vi "Manual Override Loop.vi"(0 "Current Valve State Array":refnum<vi>, 2 "Manual Valve Array":refnum<vi>[](array[refnum]), 4 "Stop Process":refnum<vi>, 6 "System Queue":refnum<vi>, 7 "N2 Valves":i32[](array[numeric]), 8 "JSON Queue":refnum<vi>, 9 "Pump Valves":i32[](array[numeric]), 10 "Locks (-)":refnum<vi>, 11 "Valves Per Reactor":i32, 12 "Debug Mode":refnum<vi>, 13 "Number of Reactors":i32, 14 "Reactor Name":string, 15 "Reactor Selector":T1(ring), 19 "Number of Shared Lines":i32) -> ()   [LabVIEW 2021]
uses:
  a8b2c1af-05a2-43ad-9eca-c9421cccccff.vi
  <vilib>/Comparison/Equal/Equal Functor/Equal Functor.lvclass
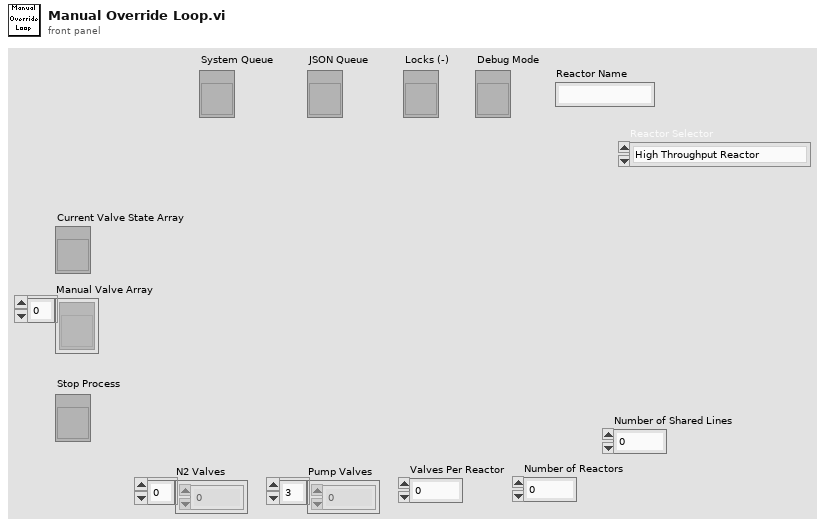
[diagram p1: front panel]
types:
  T1 = enum16{"High Throughput Reactor", "In Situ Reactor", "MLD Reactor"}
  T2 = enum16{"Lock", "Release", "Check", "Check All", "Release All"}
  T3 = enum8{"Enabled", "Disabled", "Disabled and Grayed Out"}
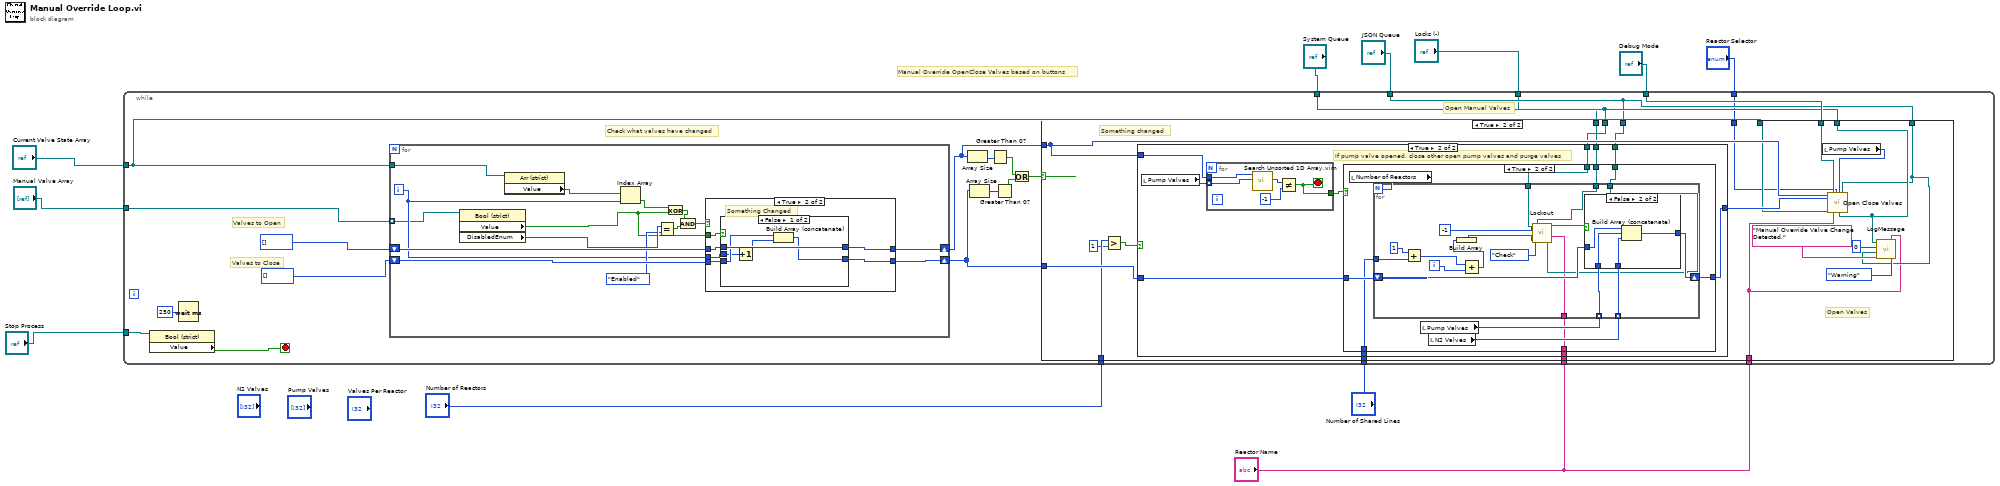
[diagram p0: block diagram]
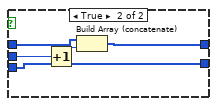
[diagram p7: hidden frame]
diagram:
  # "Manual Override OpenClose Valves based on buttons"
  n1 = while {
    tunnel: "Current Valve State Array" -> [w21]
    tunnel: "Stop Process" -> [w24]
    tunnel: "Debug Mode" -> [w22]
    tunnel: "System Queue" -> [w20]
    tunnel: "JSON Queue" -> [w19]
    tunnel: "Locks (-)" -> [w18]
    tunnel: "Manual Valve Array" -> [w17]
    tunnel: "Number of Reactors" -> [w16]
    tunnel: "Number of Shared Lines" -> [w15]
    tunnel: "Reactor Name" -> [w14]
    tunnel: "Reactor Name" -> [w13]
    tunnel: "Reactor Selector" -> [w12]
    stop <- w23 stop-if-true
    # "Open Manual Valves"
    # "Check what valves have changed"
    # "Valves to Open"
    # "Valves to Close"
    n2 = property class="Bool (strict)"(reference=w24) -> ("Value"=w23:bool)  [unwired: 1 in, 2 out]
    n3 = Wait (ms)(milliseconds to wait=u32 250 ("millisecond multiple")) -> ()  [unwired: 1 out]
    n4 = for {
      tunnel: w17 -> [w105] mode=indexing
      shift-right: [w118] -> w26
      shift-left: i32[] [] -> [w119]
      shift-right: [w116] -> w25
      shift-left: i32[] [] -> [w117]
      tunnel: w21 -> [w107]
      i -> [w108]
      n5 = property class="Bool (strict)"(reference=w105) -> ("Value"=w106:bool, "DisabledEnum"=w114:T3)  [unwired: 1 in, 2 out]
      n6 = property class="Arr (strict)"(reference=w107) -> ("Value"=w109:bool[])  [unwired: 1 in, 2 out]
      n7 = Index Array(array=w109, index=w108) -> (element=w115:bool)
      n8 = Equal?(x=w114, y=T3."Enabled") -> (x = y?=w110:bool)
      n9 = Exclusive Or(1:w106, 2:w115) -> (0:w111:bool)
      n10 = And(x=w111, y=w110) -> (x .and. y?=w112:bool)
      n11 = case shown="True" w112 {
        tunnel: w106 -> [_ w127]
        tunnel: w119 -> [w121 w126]
        tunnel: [w121 w125] -> w118
        tunnel: w108 -> [_ w124]
        tunnel: w117 -> [w120 w123]
        tunnel: [w120 w122] -> w116
        frame False {
        }
        frame True {
          # "Something Changed"
          n12 = case shown="False" w127 {
            tunnel: w126 -> [w132 w137]
            tunnel: [w132 w136] -> w125
            tunnel: w124 -> [w130 w135]
            tunnel: w123 -> [w131 w134]
            tunnel: [w129 w134] -> w122
            frame False {
              n13 = Increment(x=w130) -> (x+1=w128:i32)
              n14 = Build Array (concatenate)(w131, w128) -> (w129:i32[])
            }
            frame True {
              n15 = Increment(x=w135) -> (x+1=w133:i32)
              n16 = Build Array (concatenate)(w137, w133) -> (w136:i32[])
            }
          }
        }
      }
    }
    n17 = Array Size(array=w26) -> (size(s)=w32:i32)
    n18 = Array Size(array=w25) -> (size(s)=w29:i32)
    n19 = Greater Than 0?(x=w32) -> (x > 0?=w30:bool)
    n20 = Greater Than 0?(x=w29) -> (x > 0?=w28:bool)
    n21 = Or(x=w30, y=w28) -> (x .or. y?=w31:bool)
    n22 = case shown="True" w31 {
      tunnel: w26 -> [_ w54]
      tunnel: w25 -> [_ w53]
      tunnel: w22 -> [_ w48]
      tunnel: w20 -> [_ w47]
      tunnel: w19 -> [_ w46]
      tunnel: w21 -> [_ w45]
      tunnel: w20 -> [_ w44]
      tunnel: w19 -> [_ w43]
      tunnel: w18 -> [_ w42]
      tunnel: w16 -> [_ w40]
      tunnel: w15 -> [_ w38]
      tunnel: w14 -> [_ w36]
      tunnel: w13 -> [_ w37]
      tunnel: w12 -> [_ w35]
      frame False {
      }
      frame True {
        # "Something changed"
        # "Open Valves"
        n23 = Greater?(x=w40, y=1) -> (0:w41:bool)
        n24 = case shown="True" w41 {
          tunnel: w54 -> [_ w64]
          tunnel: w53 -> [w56 w63]
          tunnel: [w56 w62] -> w52
          tunnel: w44 -> [_ w61]
          tunnel: w43 -> [_ w60]
          tunnel: w42 -> [_ w59]
          tunnel: w38 -> [_ w58]
          tunnel: w37 -> [_ w57]
          frame False {
          }
          frame True {
            # "If pump valve opened, close other open pump valves and purge valves"
            n25 = local read "Pump Valves"() -> (w66:i32[])
            n26 = for {
              tunnel: w66 -> [w103] mode=indexing
              tunnel: w64 -> [w104]
              tunnel: [w100] -> w65
              stop <- w100 stop-if-true
              n27 = call "Search Unsorted 1D Array.vim"("element"=w103, "unsorted 1D array"=w104) -> ("index of element"=w102:i32)  [unwired: 9 in]
              n28 = Not Equal?(x=w102, y=-1) -> (x != y?=w100:bool)
            }
            n29 = case shown="True" w65 {
              tunnel: w63 -> [w67 w76]
              tunnel: [w67 w73] -> w62
              tunnel: w61 -> [_ w72]
              tunnel: w60 -> [_ w71]
              tunnel: w59 -> [_ w70]
              tunnel: w58 -> [_ w69]
              tunnel: w57 -> [_ w68]
              frame False {
              }
              frame True {
                n30 = local read "Number of Reactors"() -> (w77:i32)
                n31 = local read "Pump Valves"() -> (w75:i32[])
                n32 = local read "N2 Valves"() -> (w74:i32[])
                n33 = for {
                  N: w77 -> [_]
                  tunnel: w75 -> [w91] mode=indexing
                  tunnel: w74 -> [w90] mode=indexing
                  shift-right: [w89] -> w73
                  shift-left: w76 -> [w92]
                  tunnel: w72 -> [w84]
                  tunnel: w71 -> [w83]
                  tunnel: w70 -> [w82]
                  tunnel: w69 -> [w80]
                  tunnel: w68 -> [w78]
                  i -> [w93]
                  n34 = Add(x=1, y=w80) -> (x+y=w79:i32)
                  n35 = Add(x=w79, y=w93) -> (x+y=w94:i32)
                  n36 = Build Array(w94) -> (w87:i32[])
                  n37 = call "Lockout.vi"("Locks"=w82, "ID"=-1, "Queue System"=w84, "Request Type"=T2."Check", "Request Array"=w87, "Reactor Name"=w78, "JSON Queue"=w83) -> ("Response"=w85:bool)  [unwired: 1 out]
                  n38 = case shown="False" w85 {
                    tunnel: w92 -> [w95 w99]
                    tunnel: w91 -> [_ w98]
                    tunnel: w90 -> [_ w97]
                    tunnel: [w95 w96] -> w89
                    frame True {
                    }
                    frame False {
                      n39 = Build Array (concatenate)(w99, w98, w97) -> (w96:i32[])
                    }
                  }
                }
              }
            }
          }
        }
        n40 = local read "Pump Valves"() -> (w55:i32[])
        n41 = call "Open Close Valves.vi"("Valves to Open"=w54, "Valves to Close"=w52, "Current Valve State"=w45, "Debug Mode"=w48, "Reactor Name"=w36, "Reactor Selector"=w35, "Pump Valves"=w55, "System Queue"=w47, "JSON Queue"=w46) -> ()  [unwired: 11 in]
        n42 = call "LogMessage.vi"("Type"=enum16{"Locks", "Warning"}."Warning", "Reactor Name"=w36, "Log Entry"="Manual Override Valve Change Detected.", "System JSON Queue"=w46, "ID Number"=0, "System Queue"=w47) -> ()
      }
    }
  }
